vi "Write Arg.vi"(0 "class data in":refnum<class "MB_ENGINE.lvclass">, 5 "ARG U32":i32, 11 "error in (no error)":errorcluster) -> (4 "class data out":refnum<class "MB_ENGINE.lvclass">, 15 "error out":errorcluster)   [LabVIEW 2019, in "MB_ENGINE.lvclass"]
uses:
  MB_ENGINE.lvclass
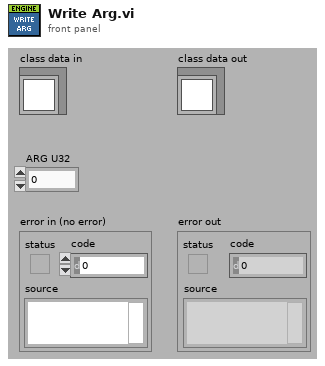
[diagram p1: front panel]
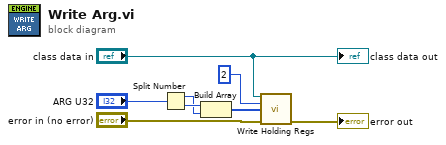
[diagram p0: block diagram]
diagram:
  n1 = Split Number(x="ARG U32") -> (hi(x)=w3:u16, lo(x)=w4:u16)
  n2 = Build Array(w4, w3) -> (w2:u16[])
  n3 = call-dynamic "Write Holding Regs.vi"("reference in"="class data in", "starting address"=u16 2, "Regs"=w2, "error in (no error)"="error in (no error)") -> ("error out"=→"error out":errorcluster)  [unwired: 11 in]
  "class data out" <- "class data in"
